vi "ReadStringSpectrum.vi"() -> ()   [LabVIEW 2009]
uses:
  tango_lv8/tango_vi.llb/ReadStringSpectrumAttribute.vi
panel:
  out "value_out":string[](array[string])
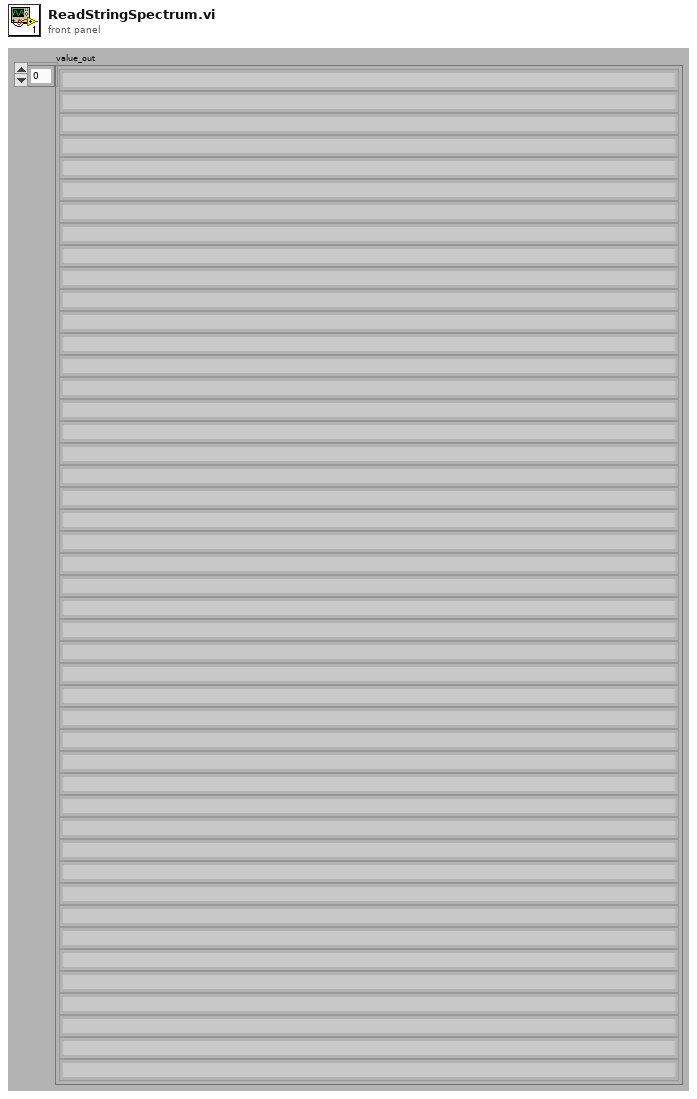
[diagram p1: front panel]
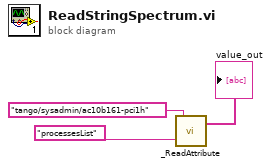
[diagram p0: block diagram]
diagram:
  n1 = call-poly "_ReadAttribute.vi"("device name"="tango/sysadmin/ac10b161-pci1h", "attribute name"="processesList") -> ("value_out"=→"value_out":string[])  [unwired: 5 out]
